vi "Main.vi"(0 "This Module":T1, 11 "error in (no error)":errorcluster) -> (15 "error out":errorcluster)   [LabVIEW 2017, in "Error Handler - Logger.lvlib"]
doc: "This VI is the Module VI containing all the code required from this Module"
uses:
  Error Handler - Logger.lvlib
  Modules.ctl
  Controls/Module - Data.ctl
  Controls/Module - States.ctl
  Controls/Timing - Data.ctl
  Controls/Process - Element.ctl
  Controls/Process.ctl
  Controls/Process - Status.ctl
  Controls/Current Error Details.ctl
  Controls/Error Types.ctl
  Controls/Timing - Mode.ctl
  Controls/Message - Queue Manager Mode.ctl
  Controls/FP - Update Value.ctl
  Controls/FP - Actionable Element.ctl
  Controls/FP - Enable_Disable.ctl
  Controls/Timing - Setup.ctl
  Controls/Message.ctl
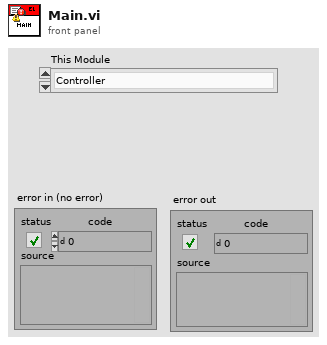
[diagram p1: front panel]
types:
  T1 = typedef "Error Handler - Logger.lvlib/Modules.ctl" = enum16{"Controller", "Error Handler - Logger"}
  T2 = typedef "Error Handler - Logger.lvlib/Message - Queue Manager Mode.ctl" = enum16{"Create", "Get", "Destroy"}
  T3 = typedef "Error Handler - Logger.lvlib/Timing - Mode.ctl" = enum16{"Reset", "Read", "Pause", "Resume"}
  T4 = typedef "Error Handler - Logger.lvlib/Module - Data.ctl" = cluster{"This Module":T1, "Current State":T5, "Timing Data":T6, "Processes":T7[], "Current Error":T10}
  T5 = typedef "Error Handler - Logger.lvlib/Module - States.ctl" = enum16{"Initialize", "Event ", "Send data", "FP Element: Update", "FP Element: Disable/Enable", "Timer: Setup", "Terminate", "--------Template----------", "Process Error", "Log ", "Log Error"}
  T6 = typedef "Error Handler - Logger.lvlib/Timing - Data.ctl" = cluster{"Elapsed Time":dbl, "Time Target":dbl, "Time Stamp":timestamp, "Paused?":bool, "Reached?":bool}
  T7 = typedef "Error Handler - Logger.lvlib/Process - Element.ctl" = cluster{"Process":T8, "Status":T9, "Data":variant}
  T8 = typedef "Error Handler - Logger.lvlib/Process.ctl" = enum16{""}
  T9 = typedef "Error Handler - Logger.lvlib/Process - Status.ctl" = enum16{"Uninitialized", "Busy"}
  T10 = typedef "Error Handler - Logger.lvlib/Current Error Details.ctl" = cluster{"Current Error Type":T11, "Error":errorcluster}
  T11 = typedef "Error Handler - Logger.lvlib/Error Types.ctl" = enum16{""}
  T12 = typedef "Error Handler - Logger.lvlib/FP - Update Value.ctl" = cluster{"FP Element":T13, "Value":string}
  T13 = typedef "Error Handler - Logger.lvlib/FP - Actionable Element.ctl" = enum16{"Put here all controls and indicators", "belonging to the UI of this module", "whose value can ", "be updated programatically", "or which can be enabled or disabled", ""}
  T14 = typedef "Error Handler - Logger.lvlib/FP - Enable_Disable.ctl" = cluster{"FP Element":T13, "Enable?":bool}
  T15 = typedef "Error Handler - Logger.lvlib/Timing - Setup.ctl" = cluster{"Mode":T3, "Update Time Target?":bool, "Time Target":dbl}
  T16 = typedef "Error Handler - Logger.lvlib/Message.ctl" = cluster{"State":T5, "Data":variant, "Originating Module":T1}
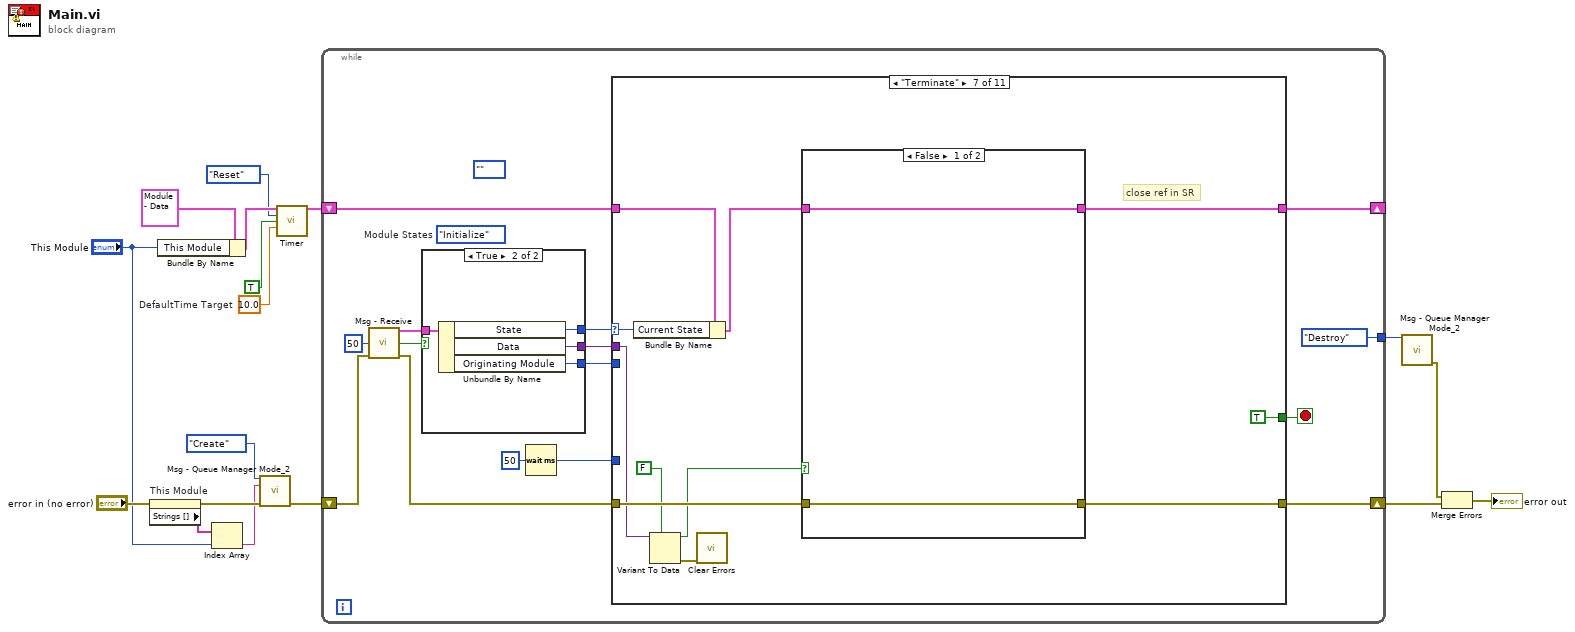
[diagram p0: block diagram]
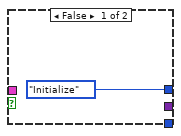
[diagram p2: hidden frame]
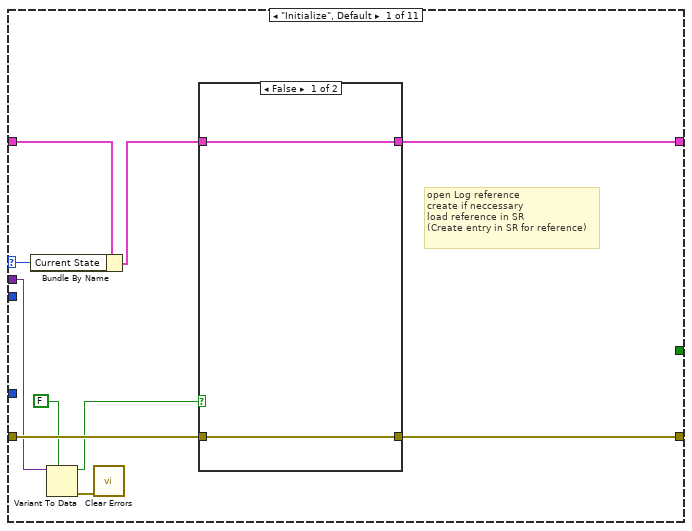
[diagram p3: hidden frame]
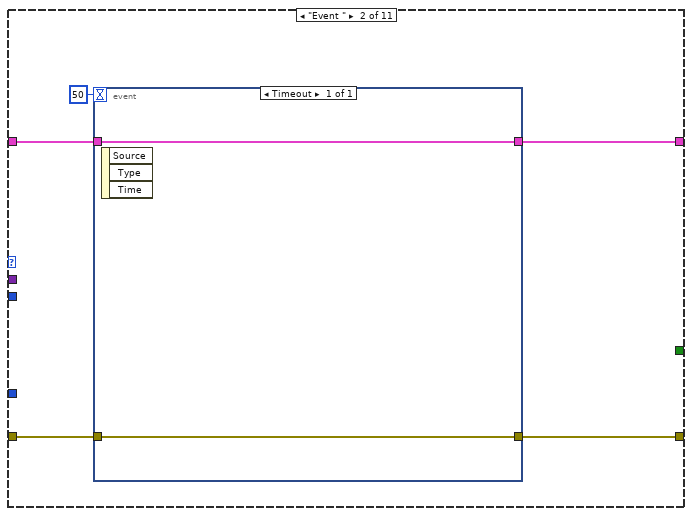
[diagram p5: hidden frame]
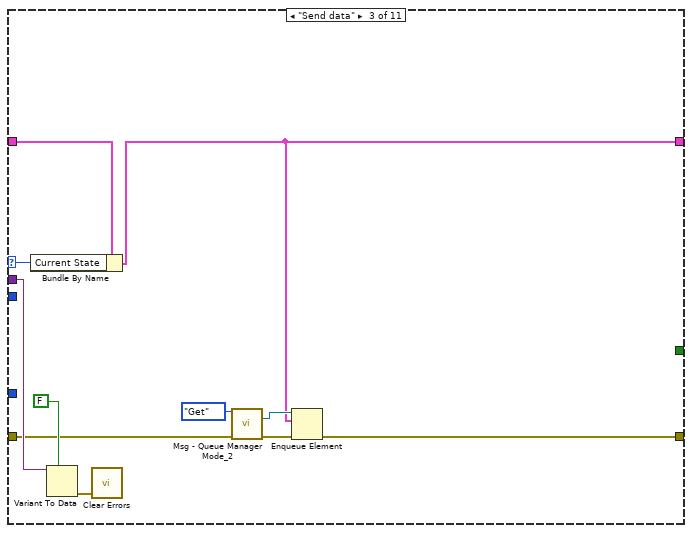
[diagram p6: hidden frame]
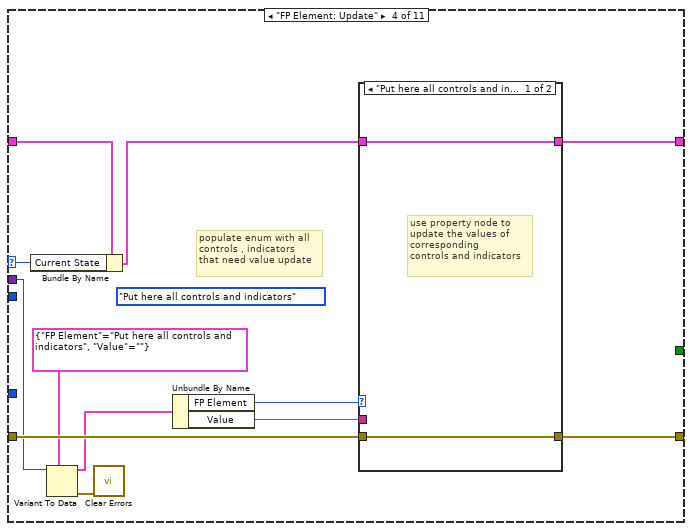
[diagram p7: hidden frame]
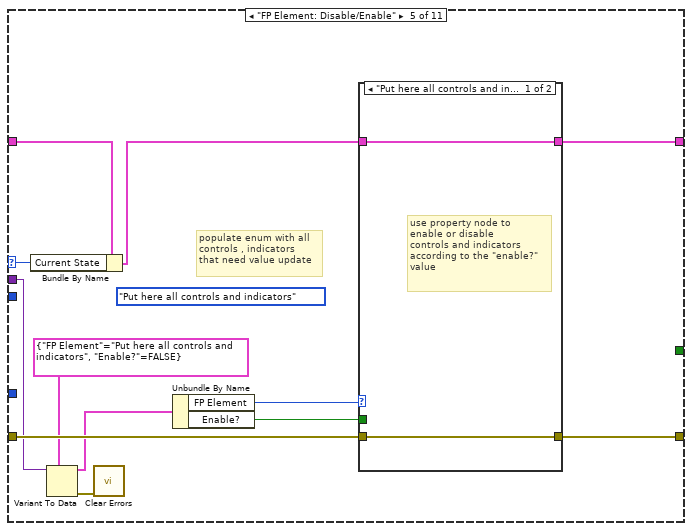
[diagram p9: hidden frame]
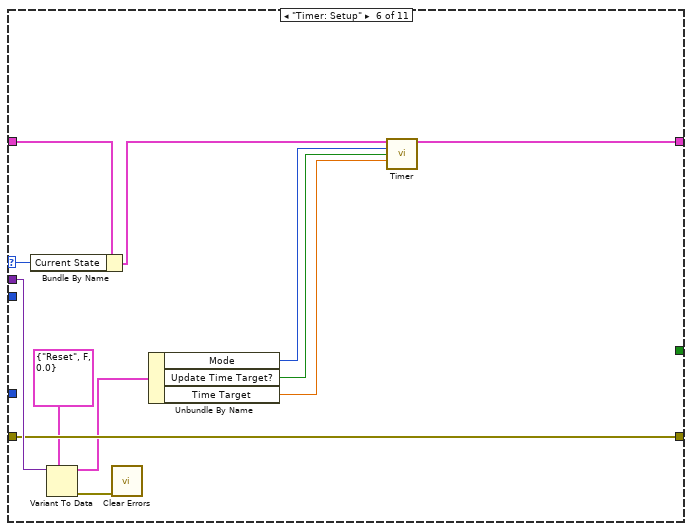
[diagram p11: hidden frame]
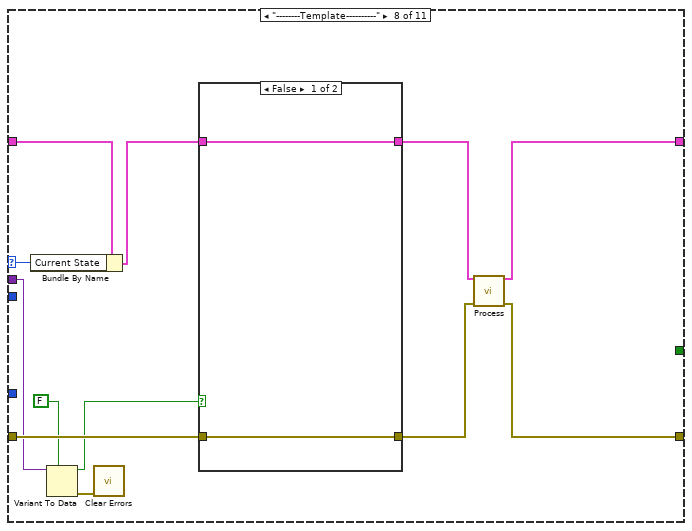
[diagram p13: hidden frame]
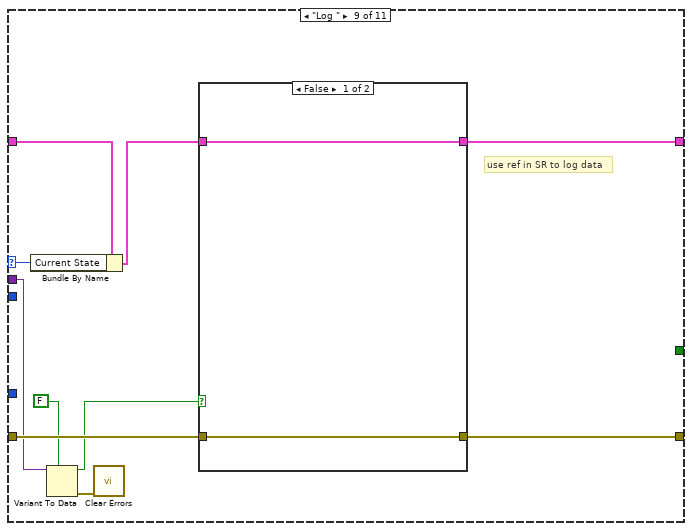
[diagram p15: hidden frame]
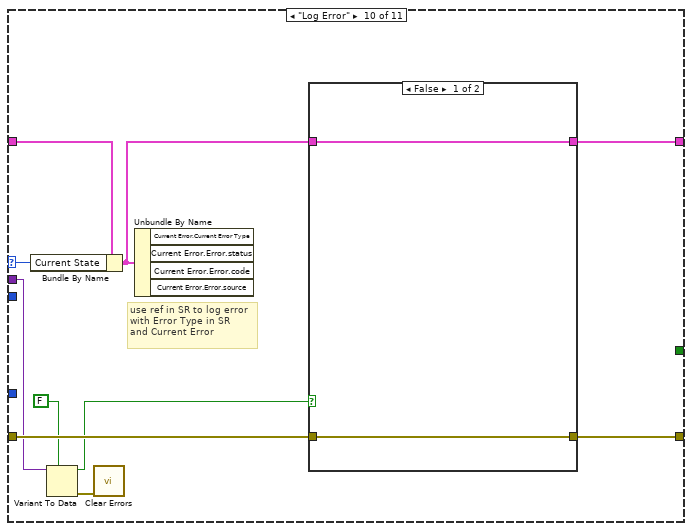
[diagram p17: hidden frame]
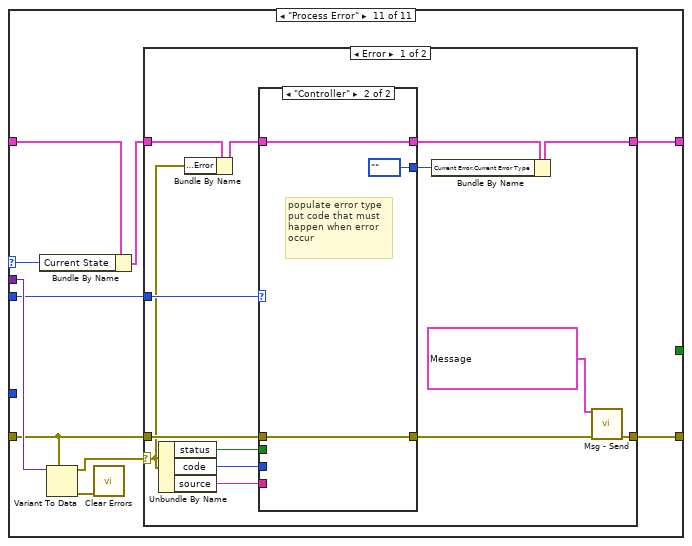
[diagram p19: hidden frame]
diagram:
  w13 = 10.0  # DefaultTime Target
  n1 = property on="This Module" class="Enum (strict)"(error in="error in (no error)") -> (error out=w8:errorcluster, "Strings []"=w10:string[])  [unwired: 1 in, 1 out]
  n2 = Bundle By Name(cluster=T4 {"This Module"=enum."Controller", "Current State"=enum."Initialize", "Timing Data"={"Elapsed Time"=0.0, "Time Target"=0.0, "Time Stamp"=timestamp(0 s since 1904-01-01), "Paused?"=FALSE, "Reached?"=FALSE}, "Processes"=[], "Current Error"={"Current Error Type"=enum."", "Error"={"status"=FALSE, "code"=0, "source"=""}}} ("Module Data In"), "This Module"="This Module") -> (w16:T4)
  n3 = Index Array(array=w10, index="This Module") -> (element=w7:string)
  n4 = call "Msg - Queue Manager Mode_2.vi"("Mode"=Message_-_Queue_Manager_Mode."Create", "Module Name"=w7, "error in (no error)"=w8) -> ("error out"=w6:errorcluster)  [unwired: 10 in, 2 out]
  n5 = call "Timer.vi"("Module Data In"=w16, "Mode"=Timing_-_Mode."Reset", "Update Target?"=TRUE, "Time Target"=w13) -> ("Module Data Out"=w15:T4)  [unwired: 8 in, 3 out]
  n6 = while {
    shift-right: [w19] -> _
    shift-left: w15 -> [w32]
    shift-right: [w31] -> w3
    shift-left: w6 -> [w29]
    tunnel: [Message_-_Queue_Manager_Mode."Destroy" ("Mode")] -> w1
    stop <- w20 stop-if-true
    (unwired) Error_Types."" ("Error Types")
    (unwired) Module_-_States."Initialize"  # Module States
    n7 = call "Msg - Receive.vi"("Timeout (ms)"=50, "error in (no error)"=w29) -> ("Message"=w25:T16, "timed out?"=w26:bool, "error out"=w28:errorcluster)  [unwired: 11 in]
    n8 = case shown="True" w26 {
      tunnel: w25 -> [_ w37]
      tunnel: [Module_-_States."Initialize" ("State") w36] -> w24
      tunnel: [_ w35] -> w23
      tunnel: [_ w34] -> w18
      frame False {
      }
      frame True {
        n9 = Unbundle By Name(w37) -> ("State"=w36:T5, "Data"=w35:variant, "Originating Module"=w34:T1)
      }
    }
    n10 = Wait (ms)(milliseconds to wait=u32 50) -> (millisecond timer value=w21:u32)
    n11 = case shown="\"Terminate\"" w24 {
      selector: w24 -> [w47 _ w69 w81 w97 w113 w124 w140 w154 w168 w182]
      tunnel: [w40 w55 w64 w76 w92 w105 w117 w133 w147 w162 w177] -> w19
      tunnel: w32 -> [w46 w54 w68 w80 w96 w112 w123 w139 w153 w167 w181]
      tunnel: [w39 w52 w62 w75 w91 w110 w116 w130 w146 w161 w176] -> w31
      tunnel: w28 -> [w44 w53 w63 w78 w94 w110 w121 w137 w151 w166 w174]
      tunnel: w23 -> [w43 _ w67 w77 w93 w111 w120 w136 w150 w165 w179]
      tunnel: w21 -> [_ _ _ _ _ _ _ _ _ _ _]
      tunnel: [_ _ _ _ _ _ TRUE _ _ _ _] -> w20
      tunnel: w18 -> [_ _ _ _ _ _ _ _ _ _ w173]
      frame "Initialize", Default {
        # "open Log reference\ncreate if neccessary\nload reference in SR\n(Create entry in SR for reference)"
        n12 = Bundle By Name(cluster=w46, "Current State"=w47) -> (w45:T4)
        n13 = Variant To Data(type=FALSE, Variant=w43) -> (data=w41:bool, error out=w38:errorcluster)  [unwired: 1 in]
        n14 = call <vilib>:"Clear Errors.vi"("error in (no error)"=w38) -> ()  [unwired: 5 in, 2 out]
        n15 = case shown="False" w41 {
          tunnel: w45 -> [w49 w51]
          tunnel: [w49 w51] -> w40
          tunnel: w44 -> [w48 w50]
          tunnel: [w48 w50] -> w39
          frame False {
          }
          frame True {
          }
        }
      }
      frame "Event " {
        n16 = event shown="[0] Timeout" {
          selector: _ -> [_]
          dyn-events: _ -> [_]
          timeout: 50 -> [_]
          tunnel: [w58] -> w55
          tunnel: w54 -> [w58]
          tunnel: w53 -> [w57]
          tunnel: [w57] -> w52
          event Timeout {
            n17 = event-data() -> ()  [unwired: 1 in, 3 out]
          }
        }
      }
      frame "Send data" {
        n18 = Bundle By Name(cluster=w68, "Current State"=w69) -> (w64:T4)
        n19 = Variant To Data(type=FALSE, Variant=w67) -> (error out=w60:errorcluster)  [unwired: 1 in, 1 out]
        n20 = call <vilib>:"Clear Errors.vi"("error in (no error)"=w60) -> ()  [unwired: 5 in, 2 out]
        n21 = call "Msg - Queue Manager Mode_2.vi"("Mode"=Message_-_Queue_Manager_Mode."Get", "error in (no error)"=w63) -> (">>Controller"=w65:refnum<queue>, "error out"=w61:errorcluster)  [unwired: 11 in, 1 out]
        n22 = Enqueue Element(queue=w65, element=w64, error in (no error)=w61) -> (error out=w62:errorcluster)  [unwired: 1 in, 2 out]
      }
      frame "FP Element: Update" {
        (unwired) FP_-_Actionable_Element."Put here all controls and indicators" ("FP Element")
        # "populate enum with all\ncontrols , indicators \nthat need value update"
        n23 = Bundle By Name(cluster=w80, "Current State"=w81) -> (w79:T4)
        n24 = Variant To Data(type=T12 {"FP Element"=enum."Put here all controls and indicators", "Value"=""} ("Message"), Variant=w77) -> (data=w72:T12, error out=w74:errorcluster)  [unwired: 1 in]
        n25 = call <vilib>:"Clear Errors.vi"("error in (no error)"=w74) -> ()  [unwired: 5 in, 2 out]
        n26 = Unbundle By Name(w72) -> ("FP Element"=w71:T13, "Value"=w70:string)
        n27 = case shown="\"Put here all controls and indicators\", Default" w71 {
          tunnel: w79 -> [w83 w85]
          tunnel: [w83 w85] -> w76
          tunnel: w78 -> [w82 w84]
          tunnel: [w82 w84] -> w75
          tunnel: w70 -> [_ _]
          frame "Put here all controls and indicators", Default {
            # "use property node to\nupdate the values of\ncorresponding\ncontrols and indicators"
          }
          frame "belonging to the UI of this module" {
          }
        }
      }
      frame "FP Element: Disable/Enable" {
        (unwired) FP_-_Actionable_Element."Put here all controls and indicators" ("FP Element")
        # "populate enum with all\ncontrols , indicators \nthat need value update"
        n28 = Bundle By Name(cluster=w96, "Current State"=w97) -> (w95:T4)
        n29 = Variant To Data(type=T14 {"FP Element"=enum."Put here all controls and indicators", "Enable?"=FALSE} ("Message"), Variant=w93) -> (data=w89:T14, error out=w90:errorcluster)  [unwired: 1 in]
        n30 = call <vilib>:"Clear Errors.vi"("error in (no error)"=w90) -> ()  [unwired: 5 in, 2 out]
        n31 = Unbundle By Name(w89) -> ("FP Element"=w88:T13, "Enable?"=w87:bool)
        n32 = case shown="\"Put here all controls and indicators\", Default" w88 {
          tunnel: w95 -> [w99 w101]
          tunnel: [w99 w101] -> w92
          tunnel: w94 -> [w98 w100]
          tunnel: [w98 w100] -> w91
          tunnel: w87 -> [_ _]
          frame "Put here all controls and indicators", Default {
            # "use property node to\nenable or disable\ncontrols and indicators\naccording to the \"enable?\"\nvalue"
          }
          frame "belonging to the UI of this module" {
          }
        }
      }
      frame "Timer: Setup" {
        n33 = Bundle By Name(cluster=w112, "Current State"=w113) -> (w106:T4)
        n34 = Variant To Data(type=T15 {"Mode"=enum."Reset", "Update Time Target?"=FALSE, "Time Target"=0.0} ("Message"), Variant=w111) -> (data=w108:T15, error out=w109:errorcluster)  [unwired: 1 in]
        n35 = call <vilib>:"Clear Errors.vi"("error in (no error)"=w109) -> ()  [unwired: 5 in, 2 out]
        n36 = Unbundle By Name(w108) -> ("Mode"=w104:T3, "Update Time Target?"=w103:bool, "Time Target"=w102:dbl)
        n37 = call "Timer.vi"("Module Data In"=w106, "Mode"=w104, "Update Target?"=w103, "Time Target"=w102) -> ("Module Data Out"=w105:T4)  [unwired: 8 in, 3 out]
      }
      frame "Terminate" {
        # "close ref in SR"
        n38 = Bundle By Name(cluster=w123, "Current State"=w124) -> (w122:T4)
        n39 = Variant To Data(type=FALSE, Variant=w120) -> (data=w118:bool, error out=w115:errorcluster)  [unwired: 1 in]
        n40 = call <vilib>:"Clear Errors.vi"("error in (no error)"=w115) -> ()  [unwired: 5 in, 2 out]
        n41 = case shown="False" w118 {
          tunnel: w122 -> [w126 w128]
          tunnel: [w126 w128] -> w117
          tunnel: w121 -> [w125 w127]
          tunnel: [w125 w127] -> w116
          frame False {
          }
          frame True {
          }
        }
      }
      frame "--------Template----------" {
        n42 = Bundle By Name(cluster=w139, "Current State"=w140) -> (w138:T4)
        n43 = Variant To Data(type=FALSE, Variant=w136) -> (data=w134:bool, error out=w129:errorcluster)  [unwired: 1 in]
        n44 = call <vilib>:"Clear Errors.vi"("error in (no error)"=w129) -> ()  [unwired: 5 in, 2 out]
        n45 = case shown="False" w134 {
          tunnel: w138 -> [w142 w144]
          tunnel: [w142 w144] -> w132
          tunnel: w137 -> [w141 w143]
          tunnel: [w141 w143] -> w131
          frame False {
          }
          frame True {
          }
        }
        n46 = call "Process.vi"("Module Data In"=w132, "error in (no error)"=w131) -> ("Module Data Out"=w133:T4, "error out"=w130:errorcluster)  [unwired: 12 in]
      }
      frame "Log " {
        # "use ref in SR to log data"
        n47 = Bundle By Name(cluster=w153, "Current State"=w154) -> (w152:T4)
        n48 = Variant To Data(type=FALSE, Variant=w150) -> (data=w148:bool, error out=w145:errorcluster)  [unwired: 1 in]
        n49 = call <vilib>:"Clear Errors.vi"("error in (no error)"=w145) -> ()  [unwired: 5 in, 2 out]
        n50 = case shown="False" w148 {
          tunnel: w152 -> [w156 w158]
          tunnel: [w156 w158] -> w147
          tunnel: w151 -> [w155 w157]
          tunnel: [w155 w157] -> w146
          frame False {
          }
          frame True {
          }
        }
      }
      frame "Log Error" {
        # "use ref in SR to log error\nwith Error Type in SR\nand Current Error"
        n51 = Bundle By Name(cluster=w167, "Current State"=w168) -> (w159:T4)
        n52 = Variant To Data(type=FALSE, Variant=w165) -> (data=w163:bool, error out=w160:errorcluster)  [unwired: 1 in]
        n53 = call <vilib>:"Clear Errors.vi"("error in (no error)"=w160) -> ()  [unwired: 5 in, 2 out]
        n54 = Unbundle By Name(w159) -> ()  [unwired: 4 out]
        n55 = case shown="False" w163 {
          tunnel: w159 -> [w170 w172]
          tunnel: [w170 w172] -> w162
          tunnel: w166 -> [w169 w171]
          tunnel: [w169 w171] -> w161
          frame False {
          }
          frame True {
          }
        }
      }
      frame "Process Error" {
        n56 = Bundle By Name(cluster=w181, "Current State"=w182) -> (w180:T4)
        n57 = Variant To Data(type=w174, Variant=w179) -> (data=w178:errorcluster, error out=w175:errorcluster)  [unwired: 1 in]
        n58 = call <vilib>:"Clear Errors.vi"("error in (no error)"=w175) -> ()  [unwired: 5 in, 2 out]
        n59 = case shown="Error" w178 {
          selector: w178 -> [w187 w202]
          tunnel: w180 -> [w188 w203]
          tunnel: [w194 w205] -> w177
          tunnel: w174 -> [w192 w204]
          tunnel: [w184 w204] -> w176
          tunnel: w173 -> [w196 _]
          frame Error {
            n60 = Unbundle By Name(w187) -> ("status"=w191:bool, "code"=w190:i32, "source"=w189:string)
            n61 = Bundle By Name(cluster=w188, "Current Error.Error"=w187) -> (w186:T4)
            n62 = case shown="\"Controller\"" w196 {
              tunnel: w186 -> [w197 w201]
              tunnel: [w197 w201] -> w195
              tunnel: [w198 w200] -> w185
              tunnel: w192 -> [w198 w200]
              tunnel: [_ Error_Types."" ("Error Types")] -> w193
              tunnel: w191 -> [_ _]
              tunnel: w190 -> [_ _]
              tunnel: w189 -> [_ _]
              frame Default {
              }
              frame "Controller" {
                # "populate error type\nput code that must\nhappen when error \noccur"
              }
            }
            n63 = Bundle By Name(cluster=w195, "Current Error.Current Error Type"=w193) -> (w194:T4)
            n64 = call "Msg - Send.vi"("Message"=T16 {"State"=enum."Log Error", "Data"=variant, "Originating Module"=enum."Error Handler - Logger"}, "error in (no error)"=w185) -> ("error out"=w184:errorcluster)  [unwired: 13 in]
          }
          frame No Error {
            n65 = Bundle By Name(cluster=w203, "Current Error.Error"=w202) -> (w205:T4)
          }
        }
      }
    }
  }
  n66 = call "Msg - Queue Manager Mode_2.vi"("Mode"=w1) -> ("error out"=w4:errorcluster)  [unwired: 12 in, 2 out]
  n67 = Merge Errors(w4, w3) -> (→"error out":errorcluster)
